vi "1.1.vi"() -> ()   [LabVIEW 2020]
panel:
  out "Boolean 8":bool
  in  "Boolean 7":bool
  out "lATCH when relesed 4":bool
  in  "Boolean 6":bool
  out "Latch when pressed":bool
  in  "Boolean 5":bool
  out "Switch until relesed 4":bool
  in  "Boolean 3":bool
  out "Switch when Relesed 3":bool
  in  "Boolean 2":bool
  out "LED 1 Switch when pressed":bool
  in  "Boolean":bool
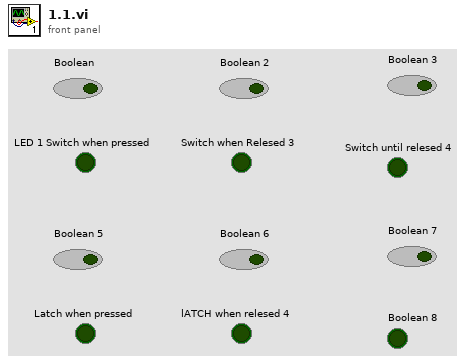
[diagram p1: front panel]
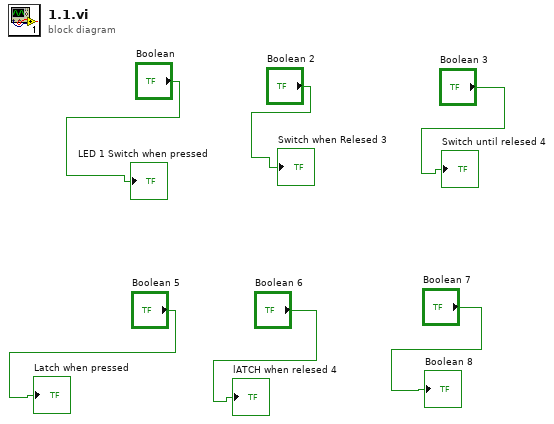
[diagram p0: block diagram]
diagram:
  "LED 1 Switch when pressed" <- "Boolean"
  "Switch when Relesed 3" <- "Boolean 2"
  "Switch until relesed 4" <- "Boolean 3"
  "Latch when pressed" <- "Boolean 5"
  "lATCH when relesed 4" <- "Boolean 6"
  "Boolean 8" <- "Boolean 7"
